vi "Word_Set_Selection_Align.vi"(5 "Word.Selection":refnum<k7>, 7 "vertical alignment":i32(ring) items=["wdCellAlignVerticalTop"=0, "wdCellAlignVerticalCenter"=1, "wdCellAlignVerticalBottom"=3], 9 "horizontal alignment":i32(ring) items=["wdAlignParagraphLeft"=0, "wdAlignParagraphCenter"=1, "wdAlignParagraphRight"=2, "wdAlignParagraphJustify"=3, "wdAlignParagraphDistribute"=4, "wdAlignParagraphJustifyMed"=5, "wdAlignParagraphJustifyHi"=7, "wdAlignParagraphJustifyLow"=8], 11 "error out 2":errorcluster) -> (15 "error out":errorcluster)   [LabVIEW 2020, in "NI_ReportGenerationToolkit.lvlib"]
uses:
  <vilib>/addons/_office/NI_ReportGenerationToolkit.lvlib
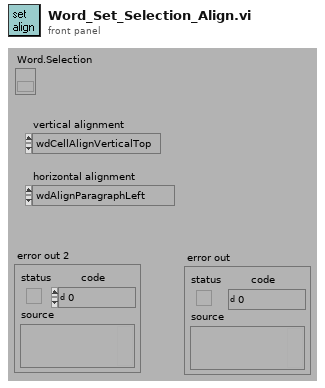
[diagram p1: front panel]
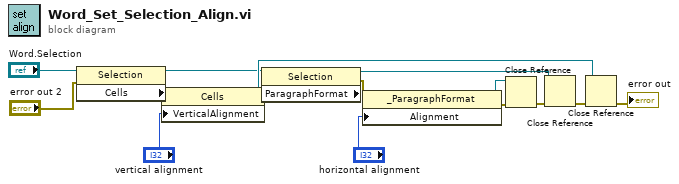
[diagram p0: block diagram]
diagram:
  n1 = property class="Selection"(reference="Word.Selection", error in="error out 2") -> (reference out=w6:refnum<k7>, error out=w5:errorcluster, "Cells"=w4:refnum<k7>)
  n2 = property class="Cells"(reference=w4, error in=w5, "VerticalAlignment"="vertical alignment") -> (reference out=w14:refnum<k7>, error out=w12:errorcluster)
  n3 = property class="Selection"(reference=w6, error in=w12) -> (reference out=w13:refnum<k7>, error out=w15:errorcluster, "ParagraphFormat"=w7:refnum<k7>)
  n4 = property class="_ParagraphFormat"(reference=w7, error in=w15, "Alignment"="horizontal alignment") -> (reference out=w11:refnum<k7>, error out=w10:errorcluster)
  n5 = Close Reference(reference=w11, error in (no error)=w10) -> (error out=w9:errorcluster)
  n6 = Close Reference(reference=w13, error in (no error)=w9) -> (error out=w8:errorcluster)
  n7 = Close Reference(reference=w14, error in (no error)=w8) -> (error out=→"error out":errorcluster)
